vi "OpenTicklish.vi"(8 "Serial USB Stimulus Port":refnum<visa-resource-name>="COM4", 11 "Use Serial USB Stimulus":bool) -> (0 "VISA resource name out":refnum<visa-resource-name>)   [LabVIEW 2015]
uses:
  <vilib>/Instr/_visa.llb/VISA Configure Serial Port (Instr).vi
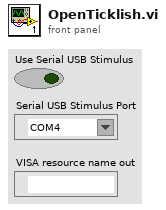
[diagram p1: front panel]
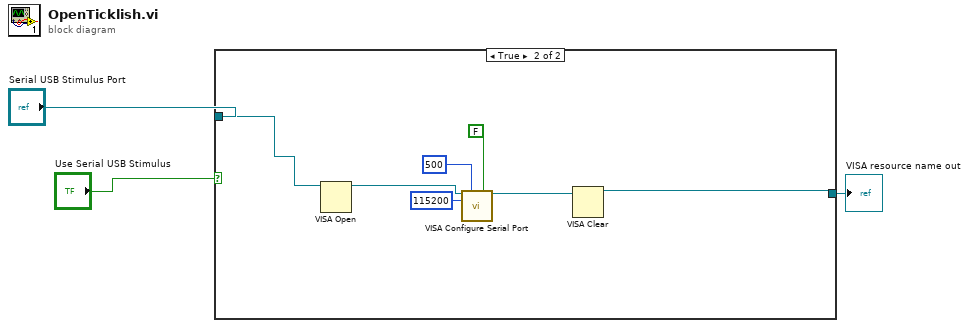
[diagram p0: block diagram]
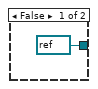
[diagram p2: hidden frame]
diagram:
  n1 = case shown="True" "Use Serial USB Stimulus" {
    tunnel: "Serial USB Stimulus Port" -> [_ w8]
    tunnel: [refnum<visa-resource-name> refnum ("VISA resource name out") w5] -> w1
    frame False {
    }
    frame True {
      n2 = VISA Open(VISA resource name=w8) -> (VISA resource name=w7:refnum<visa-resource-name>)  [unwired: 4 in, 1 out]
      n3 = call-poly "VISA Configure Serial Port"("VISA resource name"=w7, "timeout (10sec)"=u32 500, "Enable Termination\nChar (T)"=FALSE ("Enable Termination\nChar (T)"), "baud rate (9600)"=u32 115200) -> ("VISA resource name out"=w6:refnum<visa-resource-name>)  [unwired: 10 in, 1 out]
      n4 = VISA Clear(VISA resource name=w6) -> (VISA resource name out=w5:refnum<visa-resource-name>)  [unwired: 1 in, 1 out]
    }
  }
  "VISA resource name out" <- w1
